vi "Sensors BaseStation Single Value Store.vi"() -> ()   [LabVIEW 2014, in "ESP8266 WiFi Wrapper.lvlib"]
uses:
  <vilib>/Aledyne-TSXperts/Arduino Compatible Compiler for LabVIEW/addons/ESP8266 WiFi Wrapper/ESP8266 WiFi Wrapper.lvlib
  <vilib>/Aledyne-TSXperts/Arduino Compatible Compiler for LabVIEW/Arduino Compatible Compiler for LabVIEW.lvlib
panel:
  in  "DNS address":u8[](array[numeric])=[1, 2, 3, 4]
  in  "IP address":u8[](array[numeric])=[192, 168, 0, 42]
  in  "Gateway":u8[](array[numeric])=[192, 168, 0, 1]
  in  "Subnet mask":u8[](array[numeric])=[255, 255, 255, 0]
  in  "Password":string="12345678"
  in  "SSID":string="ESP8266 Wifi Example"
  in  "Listen Port":u8=80
  in  "error in (no error)":errorcluster
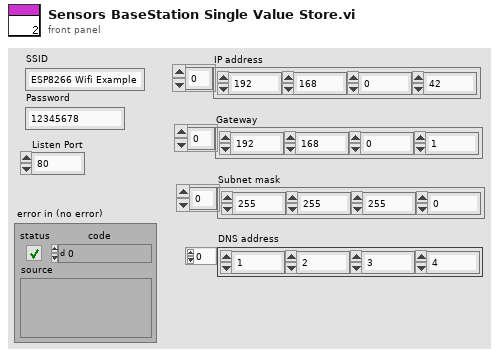
[diagram p1: front panel]
types:
  T1 = enum16{"WIFI_OFF", "WIFI_STA", "WIFI_AP", "WIFI_AP_STA"}
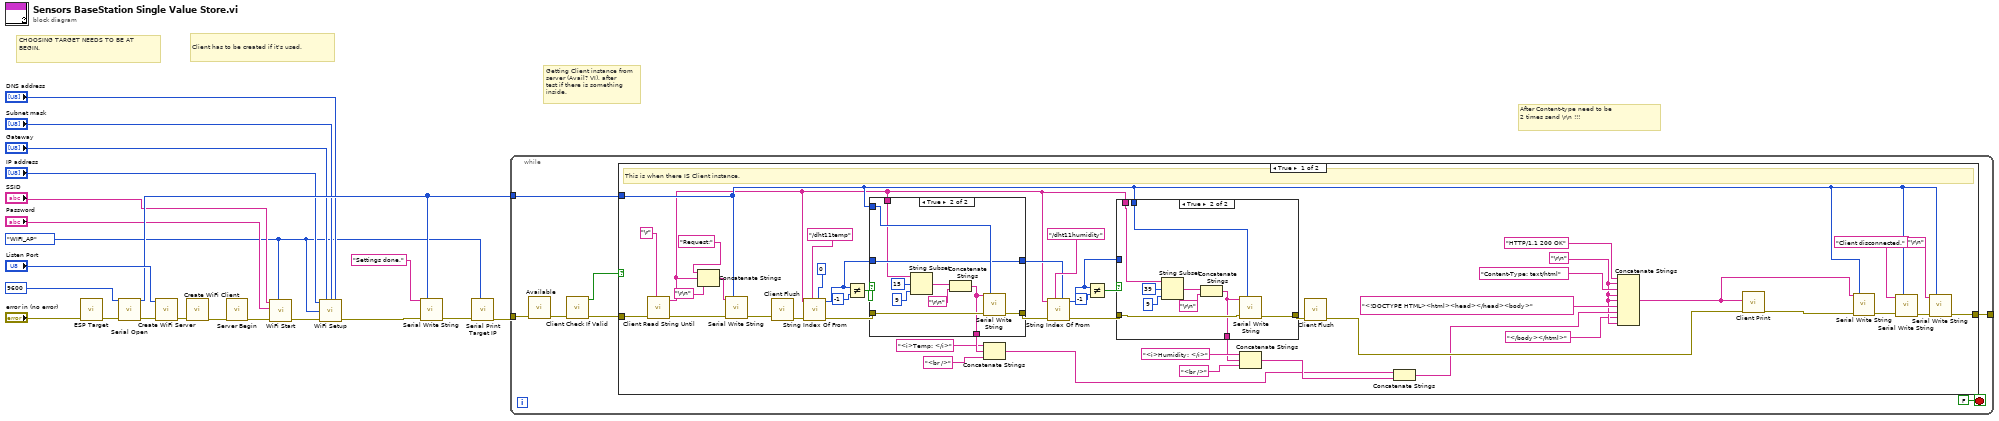
[diagram p0: block diagram]
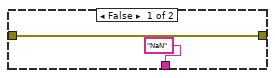
[diagram p2: hidden frame]
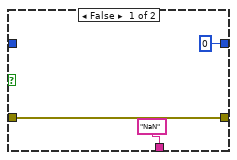
[diagram p3: hidden frame]
diagram:
  w1 = T1."WIFI_AP" ("WiFi Server Mode")
  # "After Content-type need to be\n2 times send \\r\\n !!!"
  # "Getting Client instance from\nserver (Avail? VI), after\ntest if there is something\ninside."
  # "CHOOSING TARGET NEEDS TO BE AT BEGIN."
  # "Client has to be created if it's used."
  n1 = call <vilib>:"ESP Target.vi"("Error In"="error in (no error)") -> ("Error Out"=w17:errorcluster)  [unwired: 10 in]
  n2 = call <vilib>:"Serial Open.vi"("Speed"=u32 9600, "error in (no error)"=w17) -> ("Instance"=w15:u8, "error out"=w20:errorcluster)  [unwired: 12 in]
  n3 = call <vilib>:"Create WiFi Server.vi"("Error In"=w20, "Listen Port"="Listen Port") -> ("Error Out"=w18:errorcluster)  [unwired: 9 in]
  n4 = call <vilib>:"Create WiFi Client.vi"("Error In"=w18) -> ("Error Out"=w11:errorcluster)  [unwired: 10 in]
  n5 = call <vilib>:"Server Begin.vi"("Error In"=w11) -> ("Error Out"=w13:errorcluster)  [unwired: 10 in]
  n6 = call <vilib>:"WiFi Start.vi"("WiFi Mode"=w1, "Error In"=w13, "Password"="Password", "SSID"="SSID") -> ("Error Out"=w12:errorcluster)  [unwired: 7 in]
  n7 = call <vilib>:"WiFi Setup.vi"("IP address"="IP address", "Gateway address"="Gateway", "Subnet mask"="Subnet mask", "DNS address"="DNS address", "WiFi Mode"=w1, "Error In"=w12) -> ("Error Out"=w10:errorcluster)  [unwired: 9 in]
  n8 = call <vilib>:"Serial Write String.vi"("String"="Settings done.", "Instance"=w15, "error in (no error)"=w10) -> ("error out"=w3:errorcluster)  [unwired: 12 in]
  n9 = call <vilib>:"Serial Print Target IP.vi"("WiFi Mode"=w1, "Error In"=w3) -> ("Error Out"=w2:errorcluster)  [unwired: 9 in]
  n10 = while {
    tunnel: [w26] -> _
    tunnel: w15 -> [w25]
    tunnel: w2 -> [w22]
    stop <- FALSE stop-if-true
    n11 = call <vilib>:"Available.vi"("Error In"=w22) -> ("Error Out"=w23:errorcluster)  [unwired: 10 in]
    n12 = call <vilib>:"Client Check If Valid.vi"("Error In"=w23) -> ("Error Out"=w24:errorcluster, "Is Null?"=w27:bool)  [unwired: 9 in]
    n13 = case shown="True" w27 {
      tunnel: w24 -> [w74 w99]
      tunnel: [w61 w99] -> w26
      tunnel: w25 -> [w45 _]
      frame True {
        w30 = "\r\n" ("End of Line Constant")
        # "This is when there IS Client instance."
        n14 = call <vilib>:"Client Read String Until.vi"("Terminator char"="\r" ("Carriage Return Constant"), "Error In"=w74) -> ("Error Out"=w66:errorcluster, "Read String"=w43:string)  [unwired: 8 in]
        n15 = Concatenate Strings("Request:" ("string"), w43, "\r\n" ("End of Line Constant")) -> (w60:string)
        n16 = call <vilib>:"Serial Write String.vi"("String"=w60, "Instance"=w45, "error in (no error)"=w66) -> ("error out"=w65:errorcluster)  [unwired: 12 in]
        n17 = call <vilib>:"Client Flush.vi"("Error In"=w65) -> ("Error Out"=w53:errorcluster)  [unwired: 10 in]
        n18 = call <vilib>:"String Index Of From.vi"("Start from"=u8 0, "Find string"="/dht11temp" ("IndexOf String"), "Error In"=w53, "Input String"=w43) -> ("Error Out"=w52:errorcluster, "index"=w50:i8)  [unwired: 6 in]
        n19 = Not Equal?(x=w50, y=i8 -1) -> (x != y?=w72:bool)
        n20 = case shown="True" w72 {
          tunnel: [w88 w98] -> w49
          tunnel: w52 -> [w88 w97]
          tunnel: w45 -> [_ w96]
          tunnel: w50 -> [_ w95]
          tunnel: [i8 0 ("index") w95] -> w46
          tunnel: w43 -> [_ w94]
          tunnel: ["NaN" w89] -> w42
          frame False {
          }
          frame True {
            n21 = String Subset(string=w94, offset (0)=15, length (rest)=9 ("length (rest)")) -> (substring=w91:string)
            n22 = Concatenate Strings(w91, "\r\n" ("End of Line Constant")) -> (w89:string)
            n23 = call <vilib>:"Serial Write String.vi"("String"=w89, "Instance"=w96, "error in (no error)"=w97) -> ("error out"=w98:errorcluster)  [unwired: 12 in]
          }
        }
        n24 = Concatenate Strings("<i>Temp: </i>" ("string"), w42, "<br />" ("string")) -> (w34:string)
        n25 = call <vilib>:"String Index Of From.vi"("Start from"=w46, "Find string"="/dht11humidity" ("IndexOf String"), "Error In"=w49, "Input String"=w43) -> ("Error Out"=w48:errorcluster, "index"=w44:i8)  [unwired: 6 in]
        n26 = Not Equal?(x=w44, y=i8 -1) -> (x != y?=w69:bool)
        n27 = case shown="True" w69 {
          tunnel: [w76 w85] -> w68
          tunnel: w48 -> [w76 w78]
          tunnel: w45 -> [_ w84]
          tunnel: w44 -> [_ _]
          tunnel: w43 -> [_ w79]
          tunnel: ["NaN" w77] -> w37
          frame False {
          }
          frame True {
            n28 = String Subset(string=w79, offset (0)=39, length (rest)=9 ("length (rest)")) -> (substring=w82:string)
            n29 = Concatenate Strings(w82, "\r\n" ("End of Line Constant")) -> (w77:string)
            n30 = call <vilib>:"Serial Write String.vi"("String"=w77, "Instance"=w84, "error in (no error)"=w78) -> ("error out"=w85:errorcluster)  [unwired: 12 in]
          }
        }
        n31 = Concatenate Strings("<i>Humidity: </i>" ("string"), w37, "<br />" ("string")) -> (w35:string)
        n32 = call <vilib>:"Client Flush.vi"("Error In"=w68) -> ("Error Out"=w67:errorcluster)  [unwired: 10 in]
        n33 = Concatenate Strings(w34, w35) -> (w36:string)
        n34 = Concatenate Strings("HTTP/1.1 200 OK", w30, "Content-Type: text/html", w30, w30, "<!DOCTYPE HTML><html><head></head><body>", w36, "</body></html>" ("string"), w30) -> (w56:string)
        n35 = call <vilib>:"Client Print.vi"("Error In"=w67, "Input String"=w56) -> ("Error Out"=w55:errorcluster)  [unwired: 9 in]
        n36 = call <vilib>:"Serial Write String.vi"("String"=w56, "Instance"=w45, "error in (no error)"=w55) -> ("error out"=w57:errorcluster)  [unwired: 12 in]
        n37 = call <vilib>:"Serial Write String.vi"("String"="Client disconnected.", "Instance"=w45, "error in (no error)"=w57) -> ("error out"=w64:errorcluster)  [unwired: 12 in]
        n38 = call <vilib>:"Serial Write String.vi"("String"="\r\n" ("End of Line Constant"), "Instance"=w45, "error in (no error)"=w64) -> ("error out"=w61:errorcluster)  [unwired: 12 in]
      }
      frame False {
        # "No Client instance, do nothing."
      }
    }
  }
